vi "transformacionesPosicion.vi"() -> ()   [LabVIEW 2020]
panel:
  in  "S":dbl(slide) scale=0.003..3.0
  in  "A":dbl(knob) scale=0.0..6.28
  in  "dy":dbl(slide) scale=-500.0..500.0
  in  "dx":dbl(slide) scale=-500.0..500.0
  out "new picture":picture
  in  "path to JPEG file":path=path "C:/Users/dtrej/Downloads/SVA 06 HISTOGRAMA-20250430T011009Z-001/SVA 06 HISTOGRAMA/1.jpg"
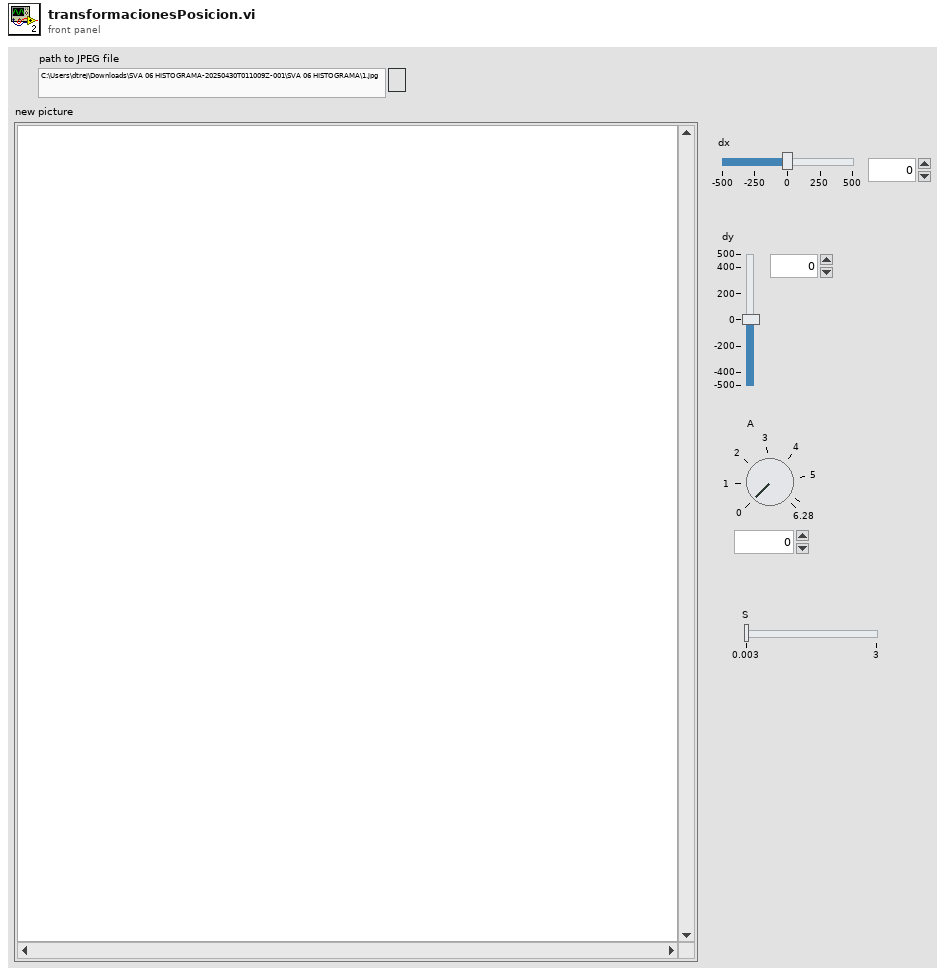
[diagram p1: front panel]
types:
  T1 = typedef "imagedata.ctl" = cluster{"image type":i32, "image depth":i32, "image":u8[], "mask":u8[], "colors":u32[], "Rectangle":cluster{"left":i16, "top":i16, "right":i16, "bottom":i16}}
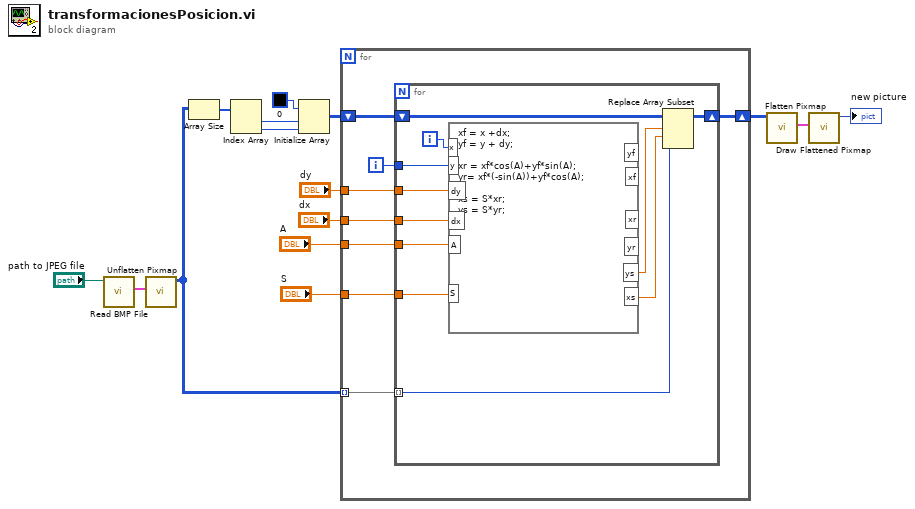
[diagram p0: block diagram]
diagram:
  n1 = call <vilib>:"Read BMP File.vi"("path to BMP file"="path to JPEG file") -> ("image data"=w14:T1)  [unwired: 8 in, 2 out]
  n2 = call <vilib>:"Unflatten Pixmap.vi"("image data"=w14) -> ("24-bit pixmap"=w11:u32[][])  [unwired: 4 in, 6 out]
  n3 = Array Size(array=w11) -> (size(s)=w10:i32[])
  n4 = Index Array(array=w10) -> (element #1=w9:i32, element #2=w8:i32)  [unwired: 2 in]
  n5 = Initialize Array(u32 0, w9, w8) -> (w6:u32[][])
  n6 = for {
    tunnel: w11 -> [w23] mode=indexing
    shift-right: [w18] -> w3
    shift-left: w6 -> [w22]
    tunnel: "dy" -> [w20]
    tunnel: "dx" -> [w19]
    tunnel: "A" -> [w17]
    tunnel: "S" -> [w16]
    i -> [w21]
    n7 = for {
      tunnel: w23 -> [w29] mode=indexing
      shift-right: [w28] -> w18
      shift-left: w22 -> [w30]
      tunnel: w21 -> [w33]
      tunnel: w20 -> [w32]
      tunnel: w19 -> [w31]
      tunnel: w17 -> [w27]
      tunnel: w16 -> [w26]
      i -> [w34]
      n8 = formula code="xf = x +dx;\nyf = y + dy;\n\nxr = xf*cos(A)+yf*sin(A);\nyr= xf*(-sin(A))+yf*cos(A);\n\nxs = S*xr;\nys = S*yr;"("x"=w34, "y"=w33, "dy"=w32, "dx"=w31, "A"=w27, "S"=w26) -> ("ys"=w25:dbl, "xs"=w24:dbl)  [unwired: 4 out]
      n9 = Replace Array Subset(array=w30, new element=w29, index (row)=w25, index (col)=w24) -> (w28:u32[][])
    }
  }
  n10 = call <vilib>:"Flatten Pixmap.vi"("24-bit pixmap"=w3) -> ("image data"=w13:T1)  [unwired: 10 in]
  n11 = call <vilib>:"Draw Flattened Pixmap.vi"("image data"=w13) -> ("new picture"=→"new picture":picture)  [unwired: 8 in]
